vi "ValueSignalLatchBooleanString.vi"(0 "VI Reference In":refnum<vi>, 2 "delimiter (>>)":string=">>", 5 "Control Path":string, 11 "error in":errorcluster) -> (4 "VI Reference Out":refnum<vi>, 15 "error out":errorcluster)   [LabVIEW 2016, in "Drona.lvlib"]
doc: "Sets the value of control which is specified. \n\nThe input control name is given as a string , incase of path, use delimiters inbetween the path."
uses:
  Drona.lvlib
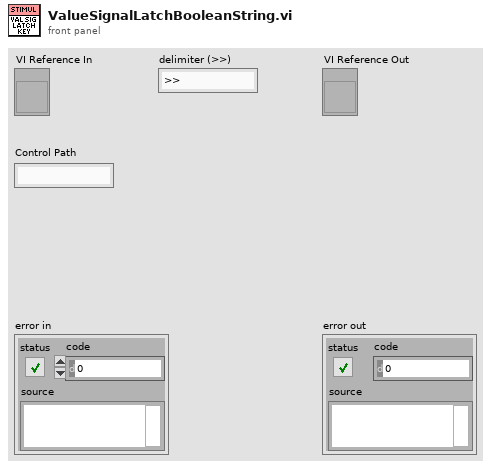
[diagram p1: front panel]
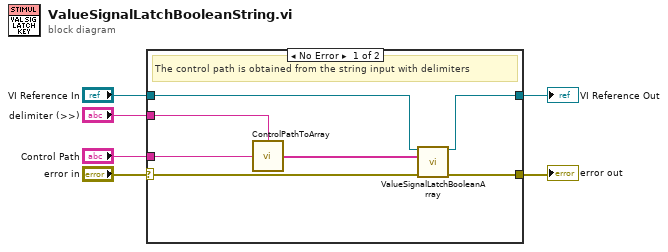
[diagram p0: block diagram]
diagram:
  n1 = case shown="No Error" "error in" {
    selector: "error in" -> [w13 w15]
    tunnel: "Control Path" -> [w9 _]
    tunnel: "VI Reference In" -> [w11 w14]
    tunnel: [w10 w14] -> w3
    tunnel: [w12 w15] -> w2
    tunnel: "delimiter (>>)" -> [w7 _]
    frame No Error {
      # "The control path is obtained from the string input with delimiters"
      n2 = call "ControlPathToArray.vi"("Control Name"=w9, "delimiter (>>)"=w7) -> ("Control Path"=w8:string[])
      n3 = call "ValueSignalLatchBooleanArray.vi"("VI Reference In"=w11, "Control Path"=w8, "error in"=w13) -> ("VI Reference Out"=w10:refnum<vi>, "error out"=w12:errorcluster)  [unwired: 11 in]
    }
    frame Error {
    }
  }
  "error out" <- w2
  "VI Reference Out" <- w3
